vi "例8.10连续输出（非重复生成)1.vi"() -> ()   [LabVIEW 2017]
uses:
  <vilib>/measure/NI_MABase.lvlib
panel:
  in  "stop (F)":bool caption="停止(F)"
  in  "sampling info":cluster{"Fs":dbl, "#s":dbl}={"Fs"=1000.0, "#s"=150.0} caption="采样信息" {"Fs" format="%.2p"}
  in  "amplitude":dbl=1.0 caption="幅值" format="%0.2p"
  in  "frequency":dbl=10.0 caption="频率" format="%0.2p"
  out "波形图":waveform(dbl)(graph)
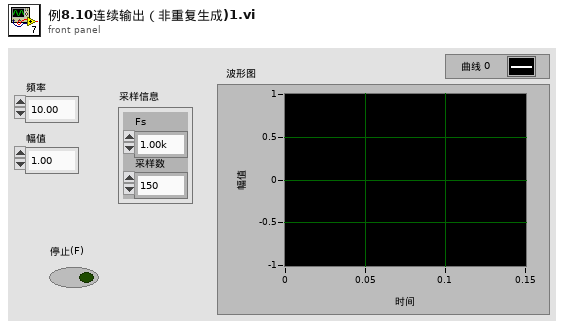
[diagram p1: front panel]
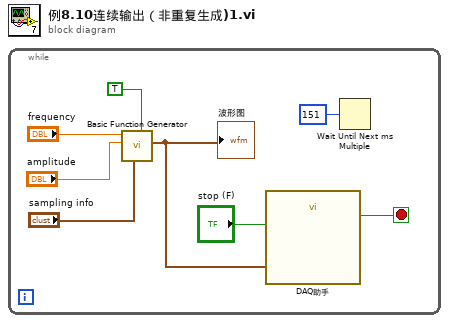
[diagram p0: block diagram]
diagram:
  n1 = while {
    stop <- w7 stop-if-true
    n2 = call <vilib>:"Basic Function Generator.vi"("reset signal"=TRUE, "sampling info"="sampling info", "amplitude"="amplitude", "frequency"="frequency") -> ("signal out"=w2:waveform(dbl))  [unwired: 5 in, 2 out]
    "波形图" <- w2
    n3 = call "DAQ助手"("data"=w2, "stop (F)"="stop (F)") -> ("stopped"=w7:bool)  [unwired: 15 in, 2 out]
    n4 = Wait Until Next ms Multiple(millisecond multiple=u32 151 ("毫秒倍数")) -> ()  [unwired: 1 out]
  }
